vi "opt_test.vi"() -> ()   [LabVIEW 2020]
uses:
  <vilib>/gmath/GlobalOptimization.llb/DE_State.ctl
  <vilib>/gmath/GlobalOptimization.llb/DE_Population.ctl
  <vilib>/gmath/GlobalOptimization.llb/DE_Settings.ctl
  <vilib>/gmath/GlobalOptimization.llb/DE_Bound Mapping Method.ctl
  <vilib>/gmath/GlobalOptimization.llb/DE_Mutation Method.ctl
  <vilib>/gmath/GlobalOptimization.llb/DE_Crossover Method.ctl
  <vilib>/gmath/GlobalOptimization.llb/DE_Stopping Criteria.ctl
  <vilib>/gmath/NI_AAL_GlobalOptimization.lvlib
panel:
  out "iteration":i32 min=1 max=200 step=1
  out "Population":cluster{dbl[], dbl[]}(graph)
  in  "Numeric":i32=2
  out "best minimum":dbl format="%_5g"
  out "F(Minimum)":dbl[](array[numeric])
  out "number of function calls":i32
  out "Ending State":T1
  in  "stopping criteria":T3={"max iterations"=50, "max function calls"=-1, "max time (sec)"=-1.0}
  in  "DE settings":T4={"population size"=10, "scale factor"=0.9, "crossover probability"=0.95, "bound mapping method"=1, "mutation method"=0, "crossover method"=0} {"crossover method" items=["Uniform", "Exponential"]; "mutation method" items=["Random", "Either Or", "Best", "Target to Best"]; "bound mapping method" items=["None", "Random between Bounds and Values", "Re-Initialize"]}
  out "Minimum":dbl[](array[numeric])
  in  "Beginning State":T1
  in  "Bounds":cluster{"Min":dbl[], "Max":dbl[]}={"Min"=[-0.277, 0.503, -0.0581, -0.0216], "Max"=[-0.237, 0.583, -0.0381, -0.0016]}
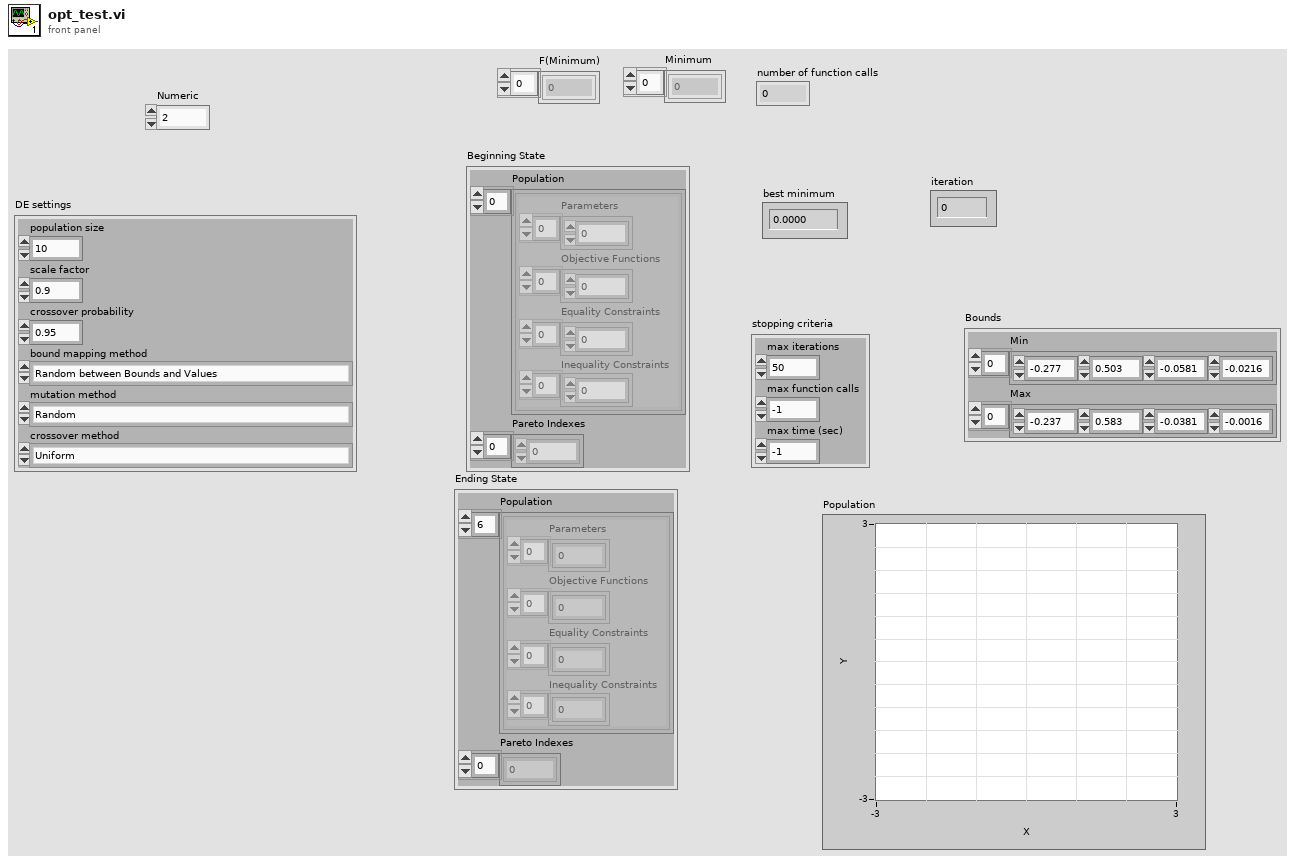
[diagram p1: front panel]
types:
  T1 = typedef "NI_AAL_GlobalOptimization.lvlib/DE_State.ctl" = cluster{"Population":T2[], "Pareto Indexes":i32[]}
  T2 = typedef "NI_AAL_GlobalOptimization.lvlib/DE_Population.ctl" = cluster{"Parameters":dbl[], "Objective Functions":dbl[], "Equality Constraints":dbl[], "Inequality Constraints":dbl[]}
  T3 = typedef "NI_AAL_GlobalOptimization.lvlib/DE_Stopping Criteria.ctl" = cluster{"max iterations":i32, "max function calls":i32, "max time (sec)":dbl}
  T4 = typedef "NI_AAL_GlobalOptimization.lvlib/DE_Settings.ctl" = cluster{"population size":i32, "scale factor":dbl, "crossover probability":dbl, "bound mapping method":T5, "mutation method":T6, "crossover method":T7}
  T5 = typedef "NI_AAL_GlobalOptimization.lvlib/DE_Bound Mapping Method.ctl" = u16
  T6 = typedef "NI_AAL_GlobalOptimization.lvlib/DE_Mutation Method.ctl" = u16
  T7 = typedef "NI_AAL_GlobalOptimization.lvlib/DE_Crossover Method.ctl" = u16
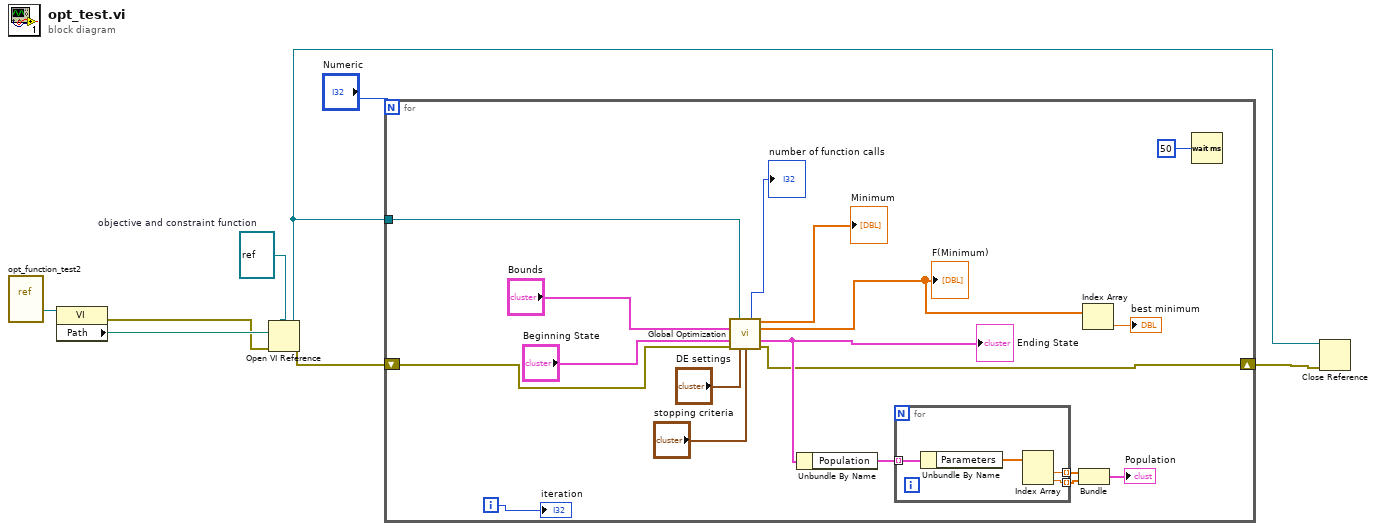
[diagram p0: block diagram]
diagram:
  w3 = refnum<vi> refnum  # objective and constraint function
  n1 = vi-ref "opt_function_test2.vi"() -> (w2:refnum<vi>)
  n2 = property class="VI"(reference=w2) -> (error out=w7:errorcluster, "Path"=w8:path)  [unwired: 1 in, 1 out]
  n3 = Open VI Reference(type specifier VI Refnum (for type only)=w3, vi path=w8, error in (no error)=w7) -> (vi reference=w5:refnum<vi>, error out=w4:errorcluster)  [unwired: 3 in]
  n4 = for {
    N: "Numeric" -> [_]
    tunnel: w5 -> [w9]
    shift-right: [w11] -> w1
    shift-left: w4 -> [w10]
    i -> [w13]
    n5 = call <vilib>:"Global Optimization.vi"("objective and constraint function"=w9, "Bounds"="Bounds", "Beginning State"="Beginning State", "error in (no error)"=w10, "DE settings"="DE settings", "stopping criteria"="stopping criteria") -> ("number of function calls"=→"number of function calls":i32, "Minimum"=→"Minimum":dbl[], "F(Minimum)"=w19:dbl[], "Ending State"=w17:T1, "error out"=w11:errorcluster)  [unwired: 5 in]
    "Ending State" <- w17
    "F(Minimum)" <- w19
    n6 = Unbundle By Name(w17) -> ("Population"=w16:T2[])
    n7 = for {
      tunnel: w16 -> [w29] mode=indexing
      tunnel: [w28] -> w15 mode=indexing
      tunnel: [w27] -> w14 mode=indexing
      n8 = Unbundle By Name(w29) -> ("Parameters"=w30:dbl[])
      n9 = Index Array(array=w30) -> (element #1=w28:dbl, element #2=w27:dbl)  [unwired: 2 in]
    }
    n10 = Bundle(w15, w14) -> (→"Population":cluster{dbl[], dbl[]})  [unwired: 1 in]
    n11 = Index Array(array=w19) -> (element=→"best minimum":dbl)  [unwired: 1 in]
    n12 = Wait (ms)(milliseconds to wait=u32 50) -> ()  [unwired: 1 out]
    "iteration" <- w13
  }
  n13 = Close Reference(reference=w5, error in (no error)=w1) -> ()  [unwired: 1 out]
